vi "niDTS Comm String Set Parameters Serial.vi"(0 "Comm String Handle":T3, 5 "Serial Resource":refnum<visa-resource-name>="COM1", 7 "Port Parameters Serial":T2={"baud rate "=115200, "data bits"=8, "Enable Termination Char"=TRUE, "flow control"=0, "parity"=enum."None", "timeout (ms) "=5000, "stop bits"=10, "termination char"=10}, 9 "CLI Login":T1, 11 "error in (no error)":errorcluster) -> (4 "Comm String Handle Out":T3, 15 "error out":errorcluster)   [LabVIEW 2014, in "niDTS CommLib.lvlib"]
doc: "This sends the Command concatenated with the Args over the String Interface.\n\nInputs:\n* Command (Required): This is the command to be sent.\n* Args (Optional): Any arguments to be concatenated with the command.\n\nOutputs:\n* Response: Any data returned from the interface. Note that no data wil be returned if the flag Read Enabled is set to FALSE."
uses:
  niDTS CommLib.lvlib
  Includes/niDTS Comm String INC Handle.ctl
  Objects/String_class/niDTS Comm String.lvclass
  Includes/niDTS Comm INC CLI Login.ctl
  Includes/niDTS Comm Serial INC Handle.ctl
  Objects/Serial_class/niDTS Comm Serial.lvclass
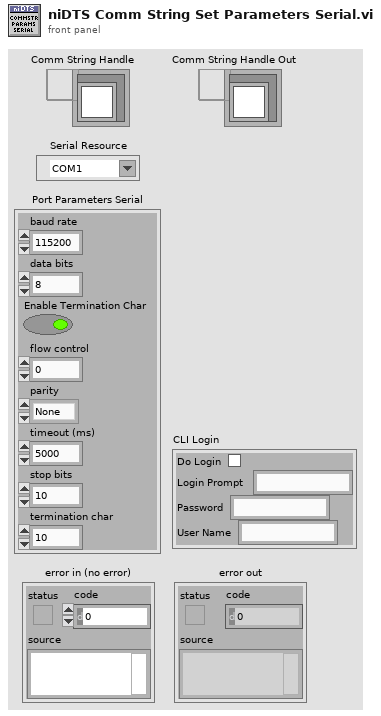
[diagram p1: front panel]
types:
  T1 = typedef "niDTS CommLib.lvlib/niDTS Comm INC CLI Login.ctl" = cluster{"Do Login":bool, "Login Prompt":string, "Password":string, "User Name":string}
  T2 = cluster{"baud rate ":u32, "data bits":u16, "Enable Termination Char":bool, "flow control":u16, "parity":enum16{"None", "Odd", "Even", "Mark", "Space"}, "timeout (ms) ":u32, "stop bits":u16, "termination char":u8}
  T3 = typedef "niDTS CommLib.lvlib/niDTS Comm String INC Handle.ctl" = refnum<data-value>
  T4 = typedef "niDTS CommLib.lvlib/niDTS Comm Serial INC Handle.ctl" = refnum<data-value>
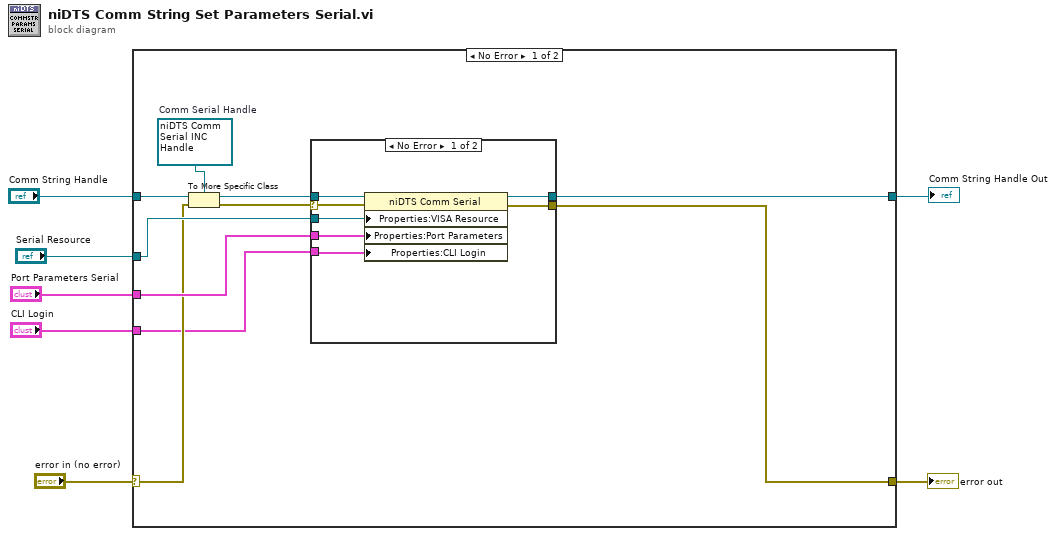
[diagram p0: block diagram]
diagram:
  n1 = case shown="No Error" "error in (no error)" {
    selector: "error in (no error)" -> [w10 w28]
    tunnel: [w9 w28] -> w7
    tunnel: "Comm String Handle" -> [w17 w27]
    tunnel: [w11 w27] -> w5
    tunnel: "Serial Resource" -> [w13 _]
    tunnel: "Port Parameters Serial" -> [w12 _]
    tunnel: "CLI Login" -> [w8 _]
    frame No Error {
      w16 = T4 refnum  # Comm Serial Handle
      n2 = To More Specific Class(target class=w16, reference=w17, error in=w10) -> (specific class reference=w14:T4, error out=w15:errorcluster)
      n3 = case shown="No Error" w15 {
        selector: w15 -> [w23 w25]
        tunnel: w14 -> [w24 w26]
        tunnel: w13 -> [w22 _]
        tunnel: w12 -> [w21 _]
        tunnel: [w20 w26] -> w11
        tunnel: [w19 w25] -> w9
        tunnel: w8 -> [w18 _]
        frame No Error {
          n4 = property class="niDTS Comm Serial"(reference=w24, error in=w23, "Properties:VISA Resource"=w22, "Properties:Port Parameters"=w21, "Properties:CLI Login"=w18) -> (reference out=w20:T4, error out=w19:errorcluster)
        }
        frame Error {
        }
      }
    }
    frame Error {
    }
  }
  "error out" <- w7
  "Comm String Handle Out" <- w5
